vi "DB Insert Array data.vi"(7 "Dtat":string[](array[string]), 8 "error in (no error)":errorcluster caption="错误输入（无错误）", 9 "columns":string[](array[string]), 10 "table":string, 11 "Connncet State":T1) -> (0 "error out":errorcluster caption="错误输出", 3 "Con Ref":T1)   [LabVIEW 2014]
uses:
  <vilib>/addons/database/NI_Database_API.lvlib
  <vilib>/addons/database/Connection.llb/Conn Execute.vi
  <vilib>/addons/database/Recordset.llb/Rec Destroy - Connection.vi
  Ctr/Conneect State.ctl
  Ctr/Constr.ctl
  <vilib>/addons/database/Connection.llb/Conn ObjectReference.ctl
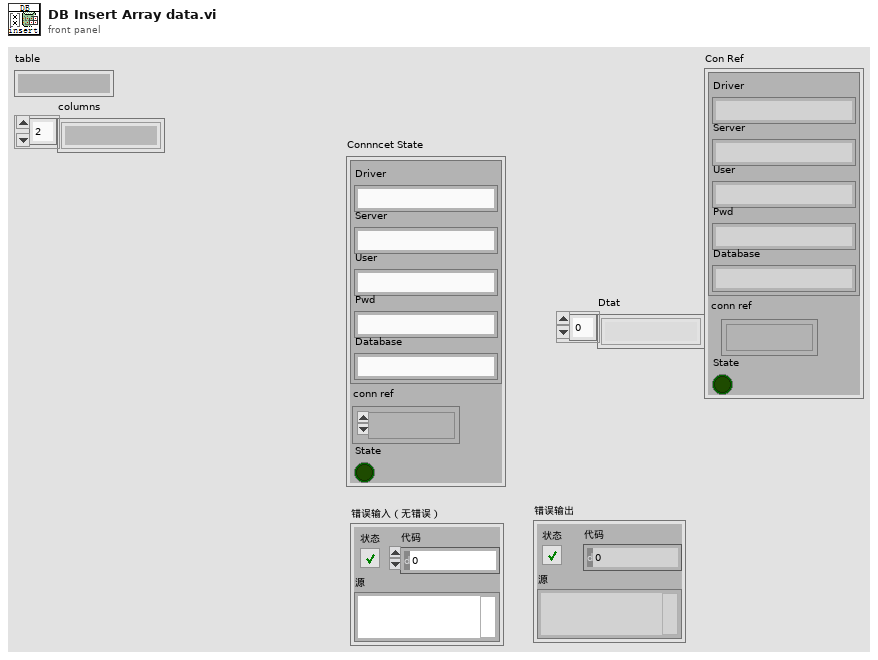
[diagram p1: front panel]
types:
  T1 = typedef "Conneect State.ctl" = cluster{"Constr":T2, "conn ref":T3, "State":bool}
  T2 = typedef "Constr.ctl" = cluster{"Driver":string, "Server":string, "User":string, "Pwd":string, "Database":string}
  T3 = typedef "NI_Database_API.lvlib/Conn ObjectReference.ctl" = refnum<k1>
  T4 = typedef "NI_Database_API.lvlib/Rec ObjectReference.ctl" = refnum<k1>
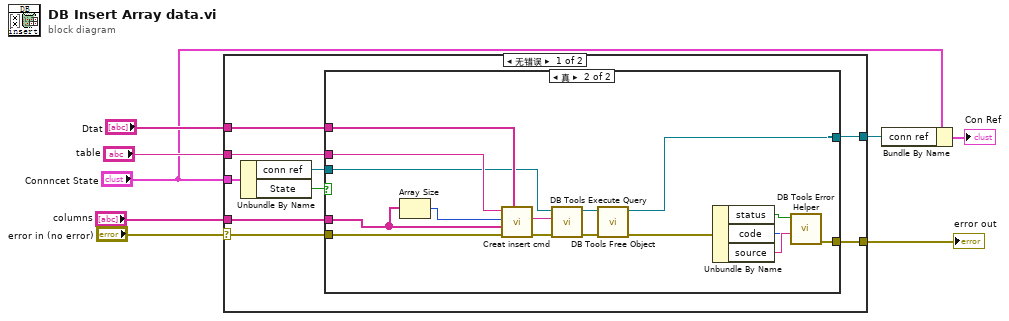
[diagram p0: block diagram]
diagram:
  n1 = case shown="无错误" "error in (no error)" {
    selector: "error in (no error)" -> [w15 w35]
    tunnel: "Connncet State" -> [w17 _]
    tunnel: "table" -> [w13 _]
    tunnel: "Dtat" -> [w12 _]
    tunnel: [w11 w35] -> w5
    tunnel: [w10 _] -> w3
    tunnel: "columns" -> [w9 _]
    frame No Error {
      n2 = Unbundle By Name(w17) -> ("conn ref"=w14:T3, "State"=w16:bool)
      n3 = case shown="真" w16 {
        tunnel: w15 -> [w18 w21]
        tunnel: w14 -> [_ w32]
        tunnel: w13 -> [_ w34]
        tunnel: w12 -> [_ w33]
        tunnel: [w18 w23] -> w11
        tunnel: [_ w22] -> w10
        tunnel: w9 -> [_ w20]
        frame False {
        }
        frame True {
          n4 = Array Size(array=w20) -> (size(s)=w19:i32)
          n5 = call "Creat insert cmd.vi"("Data"=w33, "error in (no error)"=w21, "columns"=w20, "num parameters"=w19, "table name"=w34) -> ("error out"=w30:errorcluster, "insert query"=w31:string)  [unwired: 5 in]
          n6 = call-poly <vilib>:"DB Tools Execute Query.vi"("error in (no error)"=w30, "SQL query"=w31, "connection reference"=w32) -> ("error out"=w29:errorcluster, "recordset reference"=w28:T4)  [unwired: 5 in]
          n7 = call-poly <vilib>:"DB Tools Free Object.vi"("error in (no error)"=w29, "recordset reference"=w28) -> ("error out"=w24:errorcluster, "connection reference"=w22:T3)  [unwired: 8 in]
          n8 = Unbundle By Name(w24) -> ("status"=w27:bool, "code"=w25:i32, "source"=w26:string)
          n9 = call <vilib>:"DB Tools Error Helper.vi"("source"=w26, "code"=w25, "status"=w27) -> ("error out"=w23:errorcluster)  [unwired: 8 in]
        }
      }
    }
    frame Error {
    }
  }
  "error out" <- w5
  n10 = Bundle By Name(cluster="Connncet State", "conn ref"=w3) -> (→"Con Ref":T1)
